vi "WPI_SonarMB1010AnalogRefNum Registry Get.vi"(8 "error in (no error)":errorcluster, 10 "refnum name":string="My MB1010 RefNum") -> (0 "error out":errorcluster, 3 "SonarMB1010AnalogDevRef":T1={"AIDeviceRef"={"DevStatus"={"status"=FALSE, "code"=0, "source"=""}, "Analog Channel"=enum."Invalid"}, "Scaling factor (V/in)"=0.0098, "Average Bits"=3} {"Average Bits" max=15})   [LabVIEW 2017]
doc: "Gets the reference you specify. You first must set the reference with the RefNum Registry Set VI."
uses:
  <vilib>/Rock Robotics/WPI/Ultrasonic/WPI_SonarMB1010AnalogDeviceRef.ctl
  <vilib>/Rock Robotics/WPI/AnalogChannel/WPI_AnalogChannelDevRef.ctl
  <vilib>/Rock Robotics/SystemInterfaces/AI/FPGA_AIChannel.ctl
  <vilib>/Rock Robotics/WPI/Utilities/Refnum Registry Operation.ctl
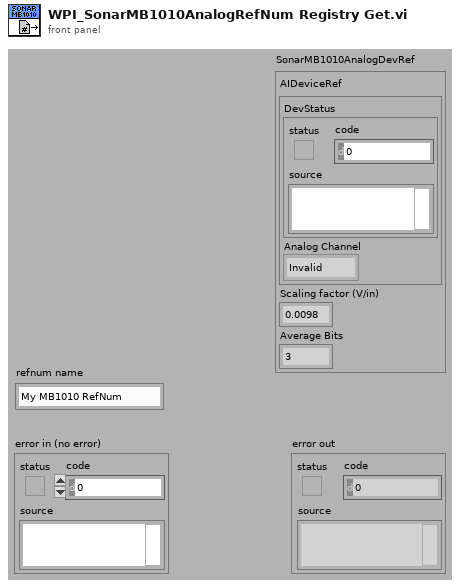
[diagram p1: front panel]
types:
  T1 = typedef "WPI_SonarMB1010AnalogDeviceRef.ctl" = cluster{"AIDeviceRef":T2, "Scaling factor (V/in)":dbl, "Average Bits":u8}
  T2 = typedef "WPI_AnalogChannelDevRef.ctl" = cluster{"DevStatus":errorcluster, "Analog Channel":T3}
  T3 = typedef "FPGA_AIChannel.ctl" = enum8{"AI 0", "AI 1", "AI 2", "AI 3", "AI MXP 0", "AI MXP 1", "AI MXP 2", "AI MXP 3", "Invalid"}
  T4 = typedef "Refnum Registry Operation.ctl" = enum16{"set", "get", "delete", "get all names", "read name"}
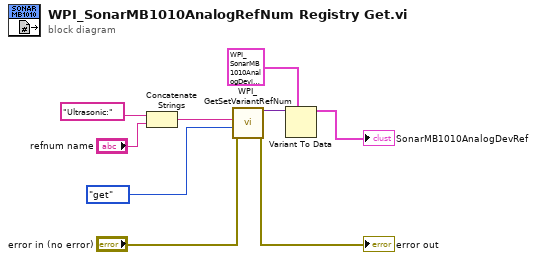
[diagram p0: block diagram]
diagram:
  n1 = Concatenate Strings("Ultrasonic:", "refnum name") -> (w9:string)
  n2 = call <vilib>:"WPI_GetSetVariantRefNum.vi"("error in (no error)"="error in (no error)", "Operation"=Refnum_Registry_Operation."get" ("menu"), "refnum name"=w9) -> ("error out"=→"error out":errorcluster, "DevRef"=w7:variant)  [unwired: 6 in, 1 out]
  n3 = Variant To Data(type=T1 {"AIDeviceRef"={"DevStatus"={"status"=FALSE, "code"=0, "source"=""}, "Analog Channel"=enum."Invalid"}, "Scaling factor (V/in)"=0.0098, "Average Bits"=3} ("SonarMB1010AnalogDevRef"), Variant=w7) -> (data=→"SonarMB1010AnalogDevRef":T1)  [unwired: 1 in, 1 out]
